vi "Get Child Bad Pointers.vi"(0 "Linked List in":refnum<class "Linked List.lvclass">, 1 "Linked List ID":string, 5 "Removed Unique ID":string, 7 "Bad Pointers":string[](array[string]), 11 "error in (no error)":errorcluster) -> (3 "Linked List ID out":string, 4 "Linked List out":refnum<class "Linked List.lvclass">, 8 "Missing GUIDs out":string[](array[string]), 15 "error out":errorcluster)   [LabVIEW 2017, in "Linked Lists.lvlib" / "Linked List.lvclass"]
uses:
  <vilib>/gpm_packages/@cs/linked-list/Source/Linked List/Linked List/Linked List.lvclass
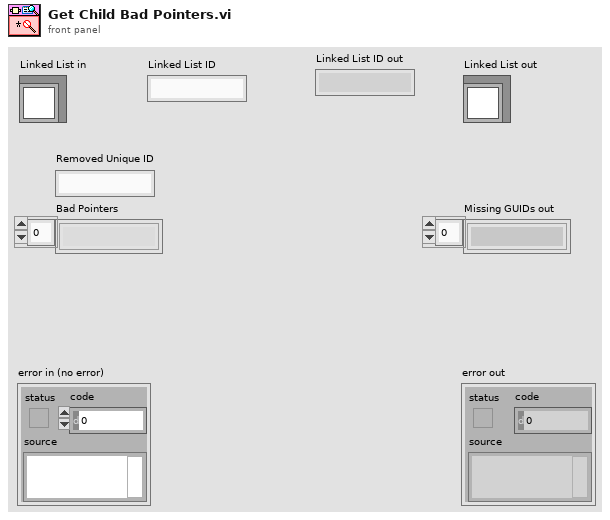
[diagram p1: front panel]
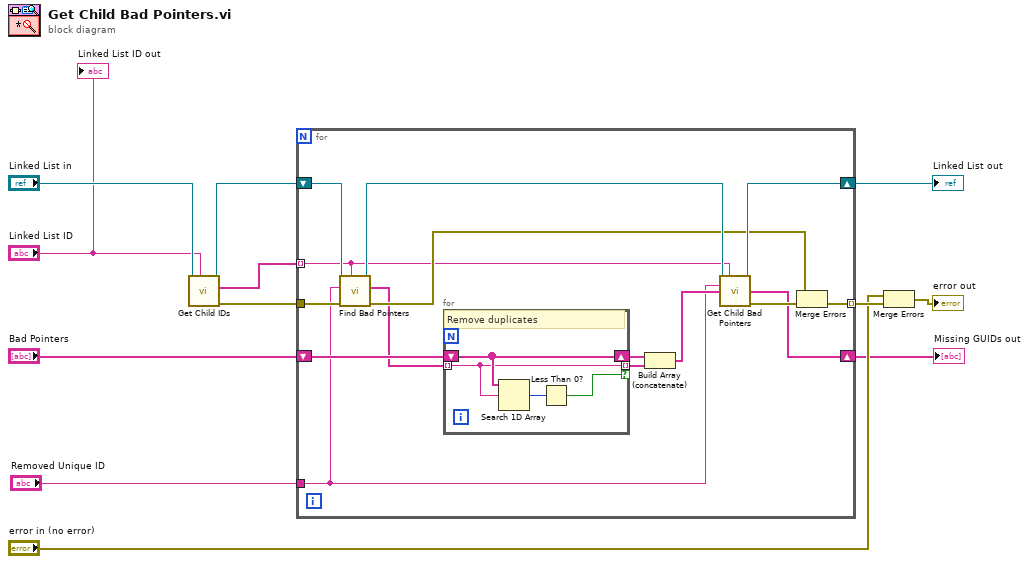
[diagram p0: block diagram]
diagram:
  n1 = call-dynamic "Get Child IDs.vi"("Linked List ID"="Linked List ID", "Linked List in"="Linked List in") -> ("error out"=w6:errorcluster, "Child IDs"=w7:string[], "Linked List out"=w8:refnum<class "Linked List.lvclass">)  [unwired: 7 in]
  n2 = for {
    shift-right: [w27] -> w10
    shift-left: w8 -> [w19]
    tunnel: w7 -> [w15] mode=indexing
    tunnel: w6 -> [w17]
    tunnel: [w25] -> w12 mode=indexing
    shift-right: [w20] -> w2
    shift-left: "Bad Pointers" -> [w24]
    tunnel: "Removed Unique ID" -> [w13]
    n3 = call <vilib>:"Find Bad Pointers.vi"("Unique ID"=w15, "error in (no error)"=w17, "Removed Unique ID"=w13, "Linked List in"=w19) -> ("error out"=w16:errorcluster, "Bad Pointers"=w14:string[], "Linked List out"=w18:refnum<class "Linked List.lvclass">)  [unwired: 5 in]
    n4 = for {
      shift-right: [w30] -> w23
      shift-left: w24 -> [w30]
      tunnel: w14 -> [w29] mode=indexing
      tunnel: [w29] -> w22 mode=indexing if=w28
      # "Remove duplicates"
      n5 = Search 1D Array(1D array=w30, element=w29) -> (index of element=w31:i32)  [unwired: 1 in]
      n6 = Less Than 0?(x=w31) -> (x < 0?=w28:bool)
    }
    n7 = Build Array (concatenate)(w23, w22) -> (w21:string[])
    n8 = call <vilib>:"Get Child Bad Pointers.vi"("Linked List in"=w18, "Linked List ID"=w15, "Removed Unique ID"=w13, "Bad Pointers"=w21) -> ("Linked List out"=w27:refnum<class "Linked List.lvclass">, "Missing GUIDs out"=w20:string[], "error out"=w26:errorcluster)  [unwired: 8 in, 1 out]
    n9 = Merge Errors(w16, w26) -> (w25:errorcluster)
  }
  "Linked List out" <- w10
  "Missing GUIDs out" <- w2
  n10 = Merge Errors("error in (no error)", w12) -> (→"error out":errorcluster)
  "Linked List ID out" <- "Linked List ID"
